vi "Summary Dialog.vi"(7 "Console Log in":refnum<class "Console Log.lvclass">, 8 "error in":errorcluster, 11 "Potting Procedure in":refnum<class "Potting Procedure.lvclass">) -> (0 "error out":errorcluster, 2 "Canceled":bool, 3 "Potting Procedure out":refnum<class "Potting Procedure.lvclass">, 5 "Console Log out":refnum<class "Console Log.lvclass">)   [LabVIEW 2011]
uses:
  Procedure Classes/Potting Procedure/Potting Procedure.lvclass
  Application Utilities/Console Log/Console Log.lvclass
  Shared Components/Config Manager Class/Type Definitions/Named Position.ctl
  Shared Components/Gantry Class/Gantry Class.lvclass
  Shared Components/Config Manager Class/Config Manager Class.lvclass
panel:
  in  "Additional Comments":string
  in  "Sylgard Batch":string
  in  "Has Database Been Updated?":enum32{"Yes", "No"}(radio)
  in  "Dispenser Input Pressure(psi)":dbl
  in  "Operator Name":string
  in  "Cancel Button":bool
  in  "OK Button":bool
  # "The potting routine has finished. \n\nPlease fill in the fields to the right, remove the syringe from \nthe holder, and press ok."
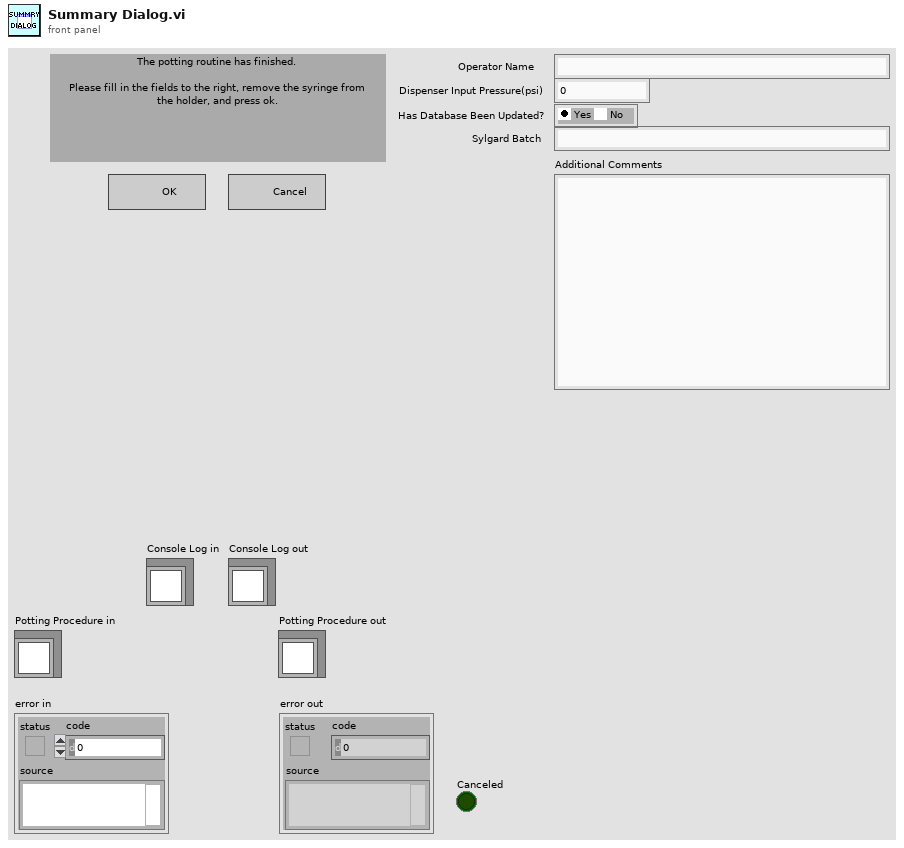
[diagram p1: front panel]
types:
  T1 = typedef "Named Position.ctl" = enum16{"home", "module_chuck_0", "module_chuck_1", "module_chuck_2", "module_chuck_3", "module_chuck_4", "glue_reservoir_chuck", "stamp_tool_chuck", "weight_tool_chuck", "needle_calibration", "tool_rack_pos_0_in", "tool_rack_pos_0_out", "tool_rack_pos_1_in", "tool_rack_pos_1_out", "tool_rack_pos_2_in", "tool_rack_pos_2_out", "front_load_position", "grabber_start_pos", "between_chuck_0_and_1", "between_chuck_2_and_3"}
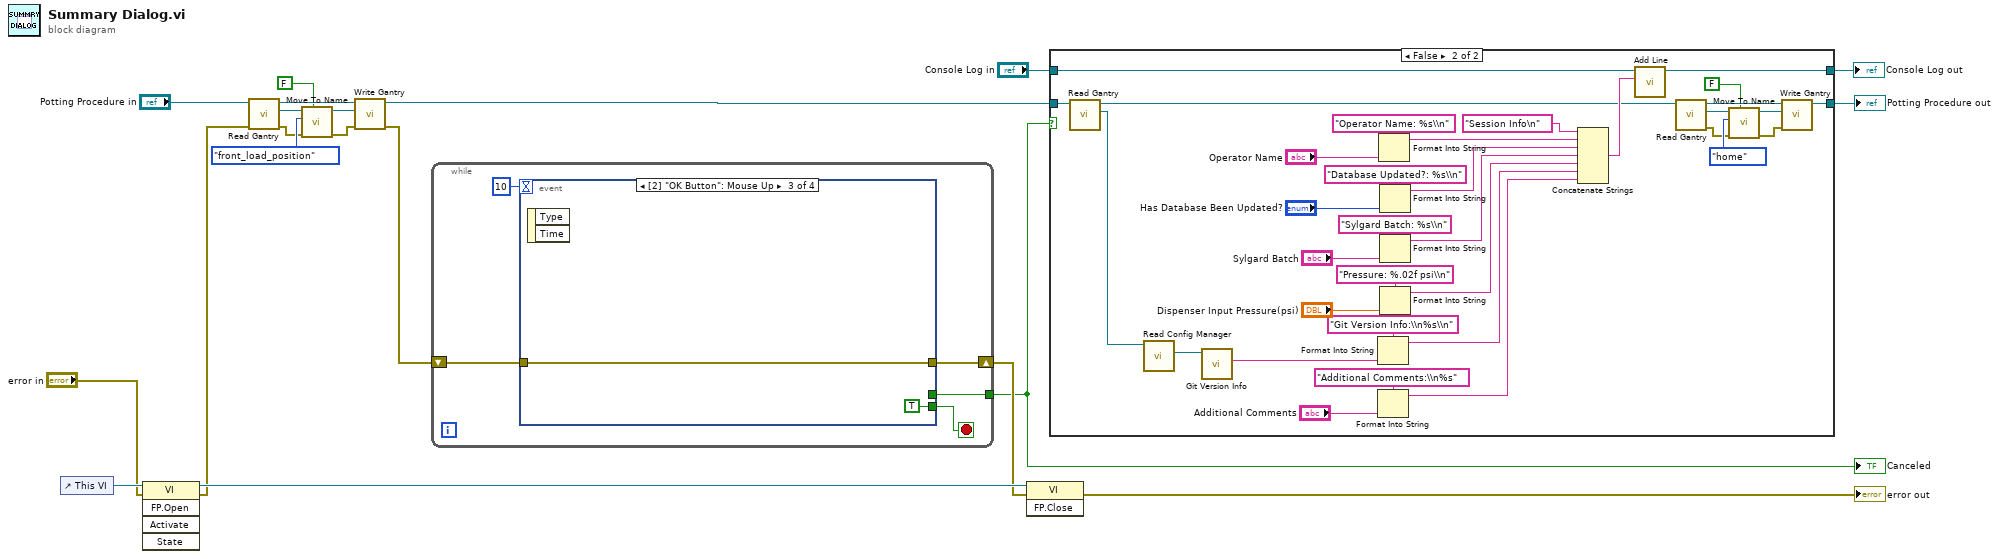
[diagram p0: block diagram]
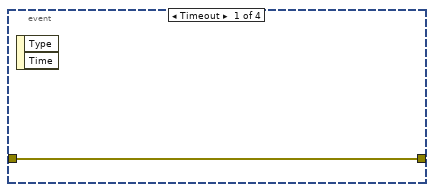
[diagram p3: hidden frame]
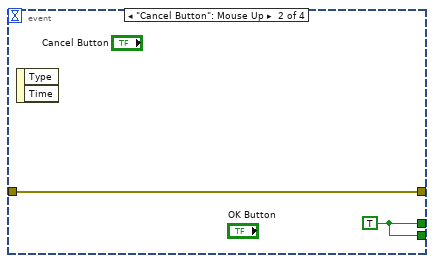
[diagram p4: hidden frame]
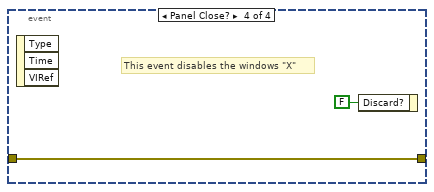
[diagram p5: hidden frame]
diagram:
  n1 = control-ref of="This VI"() -> (w20:refnum<vi>)
  n2 = invoke class="VI" method="FP.Open"(reference=w20, error in="error in") -> (reference out=w19:refnum<vi>, error out=w9:errorcluster)  [unwired: 3 in, 3 out]
  n3 = call-dynamic "Read Gantry.vi"("error in (no error)"=w9, "Potting Procedure in"="Potting Procedure in") -> ("error out"=w12:errorcluster, "Gantry"=w15:refnum<class "Gantry Class.lvclass">, "Potting Procedure out"=w11:refnum<class "Potting Procedure.lvclass">)  [unwired: 7 in]
  n4 = call-dynamic "Move To Name.vi"("Move if Same"=FALSE, "error in"=w12, "Destination"=Named_Position."front_load_position", "Gantry in"=w15) -> ("error out"=w8:errorcluster, "Gantry out"=w10:refnum<class "Gantry Class.lvclass">)  [unwired: 6 in]
  n5 = call-dynamic "Write Gantry.vi"("error in (no error)"=w8, "Gantry"=w10, "Potting Procedure in"=w11) -> ("error out"=w7:errorcluster, "Potting Procedure out"=w4:refnum<class "Potting Procedure.lvclass">)  [unwired: 7 in]
  n6 = while {
    tunnel: [w21] -> w5
    shift-right: [w23] -> w16
    shift-left: w7 -> [w22]
    stop <- w24 stop-if-true
    n7 = event shown="[2] \"OK Button\": Mouse Up" {
      selector: _ -> [_ _ _ _]
      dyn-events: _ -> [_ _ _ _]
      timeout: 10 -> [_ _ _ _]
      tunnel: [_ w27 TRUE _] -> w24
      tunnel: [w26 w28 w30 w31] -> w23
      tunnel: w22 -> [w26 w28 w30 w31]
      tunnel: [_ w27 _ _] -> w21
      event Timeout {
        n8 = event-data() -> ()  [unwired: 1 in, 2 out]
      }
      event "Cancel Button": Mouse Up {
        w27 = TRUE
        n9 = event-data() -> ()  [unwired: 1 in, 2 out]
      }
      event "OK Button": Mouse Up {
        n10 = event-data() -> ()  [unwired: 1 in, 2 out]
      }
      event Panel Close? {
        # "This event disables the windows \"X\""
        n11 = event-data() -> ()  [unwired: 1 in, 3 out]
        n12 = event-data("Discard?"=FALSE) -> ()  [unwired: 1 in, 1 out]
      }
    }
  }
  "Canceled" <- w5
  n13 = invoke class="VI" method="FP.Close"(reference=w19, error in=w16) -> (error out=→"error out":errorcluster)  [unwired: 1 in, 2 out]
  n14 = case shown="False" w5 {
    tunnel: w4 -> [w34 w42]
    tunnel: [w34 w61] -> w3
    tunnel: "Console Log in" -> [w33 w46]
    tunnel: [w33 w45] -> w1
    frame True {
    }
    frame False {
      n15 = call-dynamic "Read Gantry.vi"("Potting Procedure in"=w42) -> ("Gantry"=w40:refnum<class "Gantry Class.lvclass">, "Potting Procedure out"=w41:refnum<class "Potting Procedure.lvclass">)  [unwired: 8 in, 1 out]
      n16 = call-dynamic "Read Config Manager.vi"("Gantry in"=w40) -> ("Config Manager"=w39:refnum<class "Config Manager Class.lvclass">)  [unwired: 8 in, 2 out]
      n17 = call "Git Version Info.vi"("Config Manager in"=w39) -> ("Git Data"=w37:string)  [unwired: 8 in, 2 out]
      n18 = Format Into String(format string="Git Version Info:\\n%s\\n", w37) -> (resulting string=w35:string)  [unwired: 2 in, 1 out]
      n19 = Format Into String(format string="Additional Comments:\\n%s", "Additional Comments") -> (resulting string=w36:string)  [unwired: 2 in, 1 out]
      n20 = Format Into String(format string="Operator Name: %s\\n", "Operator Name") -> (resulting string=w50:string)  [unwired: 2 in, 1 out]
      n21 = Format Into String(format string="Database Updated?: %s\\n", "Has Database Been Updated?") -> (resulting string=w49:string)  [unwired: 2 in, 1 out]
      n22 = Format Into String(format string="Sylgard Batch: %s\\n", "Sylgard Batch") -> (resulting string=w48:string)  [unwired: 2 in, 1 out]
      n23 = Format Into String(format string="Pressure: %.02f psi\\n", "Dispenser Input Pressure(psi)") -> (resulting string=w47:string)  [unwired: 2 in, 1 out]
      n24 = Concatenate Strings("Session Info\n" ("string"), w50, w49, w48, w47, w35, w36) -> (w44:string)
      n25 = call "Add Line.vi"("String"=w44, "Console Log in"=w46) -> ("Console Log out"=w45:refnum<class "Console Log.lvclass">)  [unwired: 8 in, 1 out]
      n26 = call-dynamic "Read Gantry.vi"("Potting Procedure in"=w41) -> ("error out"=w66:errorcluster, "Gantry"=w68:refnum<class "Gantry Class.lvclass">, "Potting Procedure out"=w65:refnum<class "Potting Procedure.lvclass">)  [unwired: 8 in]
      n27 = call-dynamic "Move To Name.vi"("Move if Same"=FALSE, "error in"=w66, "Destination"=Named_Position."home", "Gantry in"=w68) -> ("error out"=w63:errorcluster, "Gantry out"=w64:refnum<class "Gantry Class.lvclass">)  [unwired: 6 in]
      n28 = call-dynamic "Write Gantry.vi"("error in (no error)"=w63, "Gantry"=w64, "Potting Procedure in"=w65) -> ("Potting Procedure out"=w61:refnum<class "Potting Procedure.lvclass">)  [unwired: 7 in, 1 out]
    }
  }
  "Potting Procedure out" <- w3
  "Console Log out" <- w1
